vi "Penel updating.vi"(1 "Action(GET)":enum16{"GET", "SET"}(ring), 7 "Panel updating in":bool, 11 "error in (no error)":errorcluster, 12 "Index(0)":i32) -> (8 "Panel updating out":bool, 15 "error out":errorcluster)   [LabVIEW 2011]
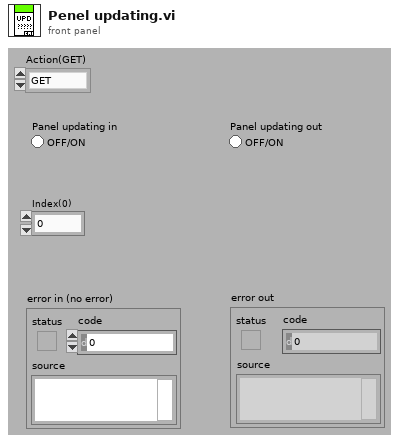
[diagram p1: front panel]
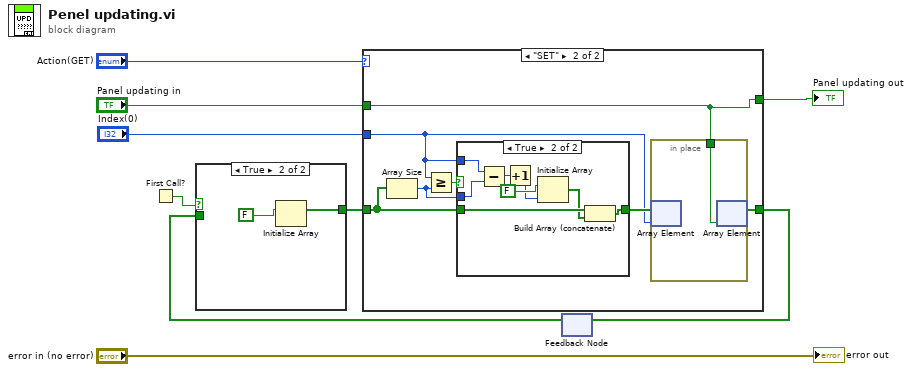
[diagram p0: block diagram]
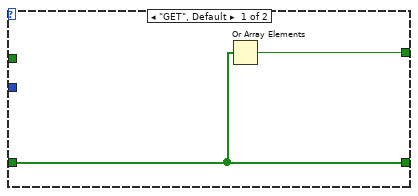
[diagram p3: hidden frame]
diagram:
  n1 = First Call?() -> (First Call?: T/F=w6:bool)
  n2 = feedback #1() -> (w7:bool[])  [unwired: 1 in]
  n3 = case shown="True" w6 {
    tunnel: w7 -> [w10 _]
    tunnel: [w10 w12] -> w4
    frame False {
    }
    frame True {
      n4 = Initialize Array(FALSE ("Panel updating")) -> (w12:bool[])  [unwired: 1 in]
    }
  }
  n5 = case shown="\"SET\"" "Action(GET)" {
    tunnel: [w14 w18] -> w5
    tunnel: w4 -> [w14 w21]
    tunnel: "Panel updating in" -> [_ w15]
    tunnel: "Index(0)" -> [_ w17]
    tunnel: [w13 w15] -> w1
    frame "GET", Default {
      n6 = Or Array Elements(Boolean array=w14) -> (logical OR=w13:bool)
    }
    frame "SET" {
      n7 = Array Size(array=w21) -> (size(s)=w16:i32)
      n8 = Greater Or Equal?(x=w17, y=w16) -> (x >= y?=w20:bool)
      n9 = case shown="True" w20 {
        tunnel: w21 -> [w23 w31]
        tunnel: [w23 w25] -> w19
        tunnel: w17 -> [_ w30]
        tunnel: w16 -> [_ w29]
        frame False {
        }
        frame True {
          n10 = Subtract(x=w30, y=w29) -> (x-y=w28:i32)
          n11 = Increment(x=w28) -> (x+1=w26:i32)
          n12 = Initialize Array(FALSE ("Panel updating"), w26) -> (w24:bool[])
          n13 = Build Array (concatenate)(w31, w24) -> (w25:bool[])
        }
      }
      n14 = in-place {
        in-place-border: w15 -> [w22]
        n15 = in-place-array #2(w19, w17) -> ()  [unwired: 1 out]
        n16 = in-place-array #2(w22) -> (w18:bool[])  [unwired: 1 out]
      }
    }
  }
  "Panel updating out" <- w1
  n17 = feedback-in #1(w5) -> ()
  "error out" <- "error in (no error)"
